vi "Calib_Inst_ch_info.vi"(1 "Input string":string) -> (0 "instrument to calibrate (new)":T1=[{"high limit (10V)"=5.0, "low limit (-10V)"=3.0, "Ch No"=1, "Off ch no"=1, "DAQmx Channel"=""}, {"high limit (10V)"=5.0, "low limit (-10V)"=3.0, "Ch No"=2, "Off ch no"=1, "DAQmx Channel"=""}] {"Off ch no" min=0 max=1; "Ch No" min=0 max=1000; "low limit (-10V)" min=-10 max=10 format="%.3f"; "high limit (10V)" min=-10 max=10 format="%.3f"})   [LabVIEW 2013]
uses:
  Controls/Calibration.ctl
panel:
  out "instrument to calibrate":T2(array[cluster])=[{"high limit (10V)"=5.0, "low limit (-10V)"=3.0, "Ch No"=1, "Off ch no"=1}, {"high limit (10V)"=5.0, "low limit (-10V)"=3.0, "Ch No"=2, "Off ch no"=1}] {"Off ch no" min=0 max=1; "Ch No" min=0 max=7; "low limit (-10V)" min=-10 max=10 format="%.3f"; "high limit (10V)" min=-10 max=10 format="%.3f"}
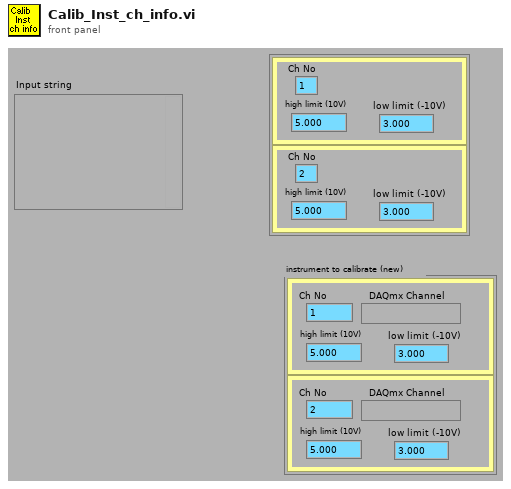
[diagram p1: front panel]
types:
  T1 = typedef "Calibration.ctl" = cluster{"high limit (10V)":sgl, "low limit (-10V)":sgl, "Ch No":i16, "Off ch no":i8, "DAQmx Channel":tag}[]
  T2 = cluster{"high limit (10V)":sgl, "low limit (-10V)":sgl, "Ch No":i16, "Off ch no":i8}[]
  T3 = cluster{"high limit (10V)":sgl, "low limit (-10V)":sgl, "Ch No":i16, "Off ch no":i8, "DAQmx Channel":tag}
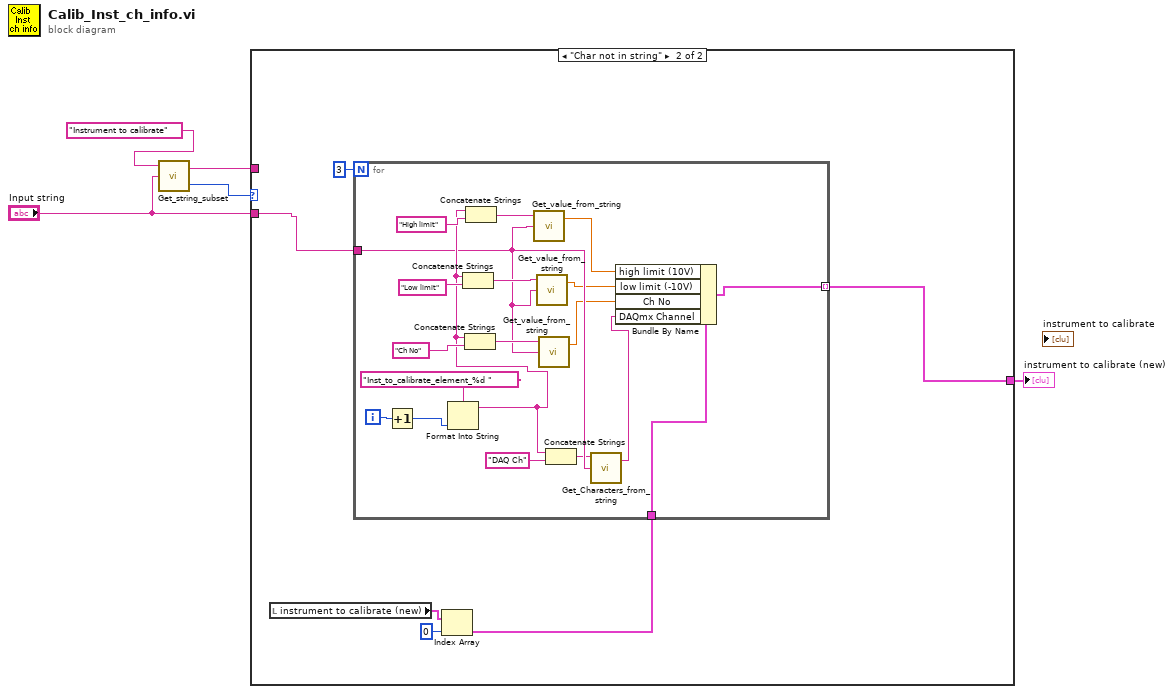
[diagram p0: block diagram]
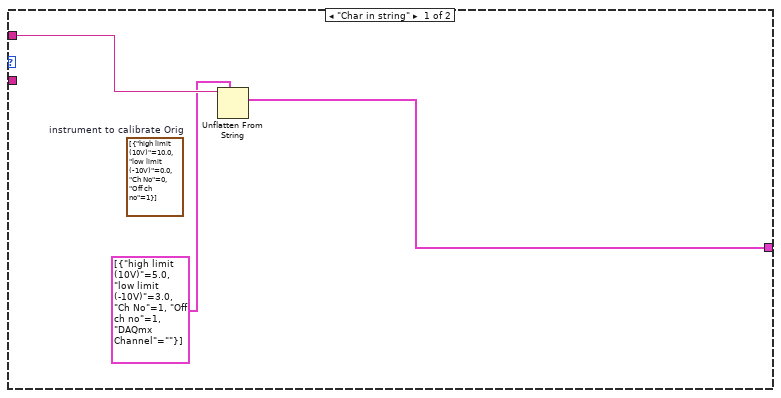
[diagram p2: hidden frame]
diagram:
  n1 = call "Get_string_subset.vi"("String to split"="Input string", "File Label"="Instrument to calibrate") -> ("Status"=w3:enum16{"Char in string", "Char not in string"}, "Output string"=w2:string)  [unwired: 2 in]
  n2 = case shown="\"Char not in string\"" w3 {
    tunnel: "Input string" -> [_ w12]
    tunnel: w2 -> [w8 _]
    tunnel: [w7 w11] -> w1
    frame "Char in string" {
      (unwired) T2 [{"high limit (10V)"=10.0, "low limit (-10V)"=0.0, "Ch No"=0, "Off ch no"=1}]  # instrument to calibrate Orig
      n3 = Unflatten From String(type=T1 [{"high limit (10V)"=5.0, "low limit (-10V)"=3.0, "Ch No"=1, "Off ch no"=1, "DAQmx Channel"=""}] ("instrument to calibrate 2"), binary string=w8) -> (value=w7:T1)  [unwired: 1 in, 4 out]
    }
    frame "Char not in string" {
      n4 = local read "instrument to calibrate (new)"() -> (w9:T1)
      n5 = Index Array(array=w9, index=0) -> (element=w13:T3)
      n6 = for {
        N: 3 -> [_]
        tunnel: w13 -> [w15]
        tunnel: w12 -> [w23]
        tunnel: [w22] -> w11 mode=indexing
        i -> [w33]
        n7 = Increment(x=w33) -> (x+1=w29:i32)
        n8 = Format Into String(format string="Inst_to_calibrate_element_%d ", w29) -> (resulting string=w27:string)  [unwired: 2 in, 1 out]
        n9 = Concatenate Strings(w27, "Low limit") -> (w24:string)
        n10 = Concatenate Strings(w27, "Ch No") -> (w25:string)
        n11 = Concatenate Strings(w27, "High limit") -> (w26:string)
        n12 = call "Get_value_from_string.vi"("Input string"=w23, "Variable name"=w26) -> ("Value"=w19:dbl)  [unwired: 1 in, 1 out]
        n13 = call "Get_value_from_string.vi"("Input string"=w23, "Variable name"=w24) -> ("Value"=w21:dbl)  [unwired: 1 in, 1 out]
        n14 = call "Get_value_from_string.vi"("Input string"=w23, "Variable name"=w25) -> ("Value"=w20:dbl)  [unwired: 1 in, 1 out]
        n15 = Concatenate Strings(w27, "DAQ Ch") -> (w17:string)
        n16 = call "Get_Characters_from_string.vi"("Input string"=w23, "Variable name"=w17) -> ("Value"=w18:string)  [unwired: 1 in, 1 out]
        n17 = Bundle By Name(cluster=w15, "high limit (10V)"=w19, "low limit (-10V)"=w21, "Ch No"=w20, "DAQmx Channel"=w18) -> (w22:T3)
      }
    }
  }
  "instrument to calibrate (new)" <- w1
